vi "GetExcelWorkSheetIndexWithName.vi"(8 "error in":errorcluster, 11 "Path":path=path "O:/Monitor/m100schedule/history/1023MT人力配置AT機台排程.xls") -> (0 "error out":errorcluster, 2 "Sheets":string[](array[string]))   [LabVIEW 2012]
doc: "Before runnig this vi you need to select the sheet and the cell you want to retrieve in LabVIEW. When you start this vi, LabVIEW will ask you the name of the Excel file. This vi was written with Excel from MS Office 97. If you edit this VI and do not have this exact version of Excel registered correctly you will get a broken arrow due to the difference in ActiveX method among Excel version. Make sure you make a copy of this vi before editing it."
panel:
  out "index of element":i32
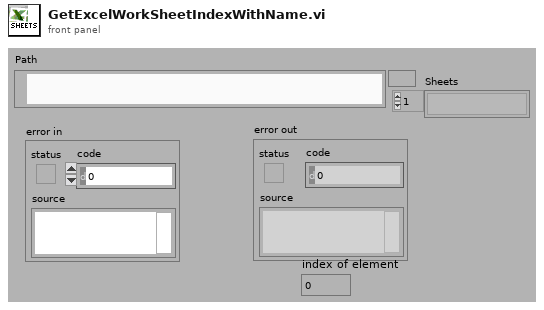
[diagram p1: front panel]
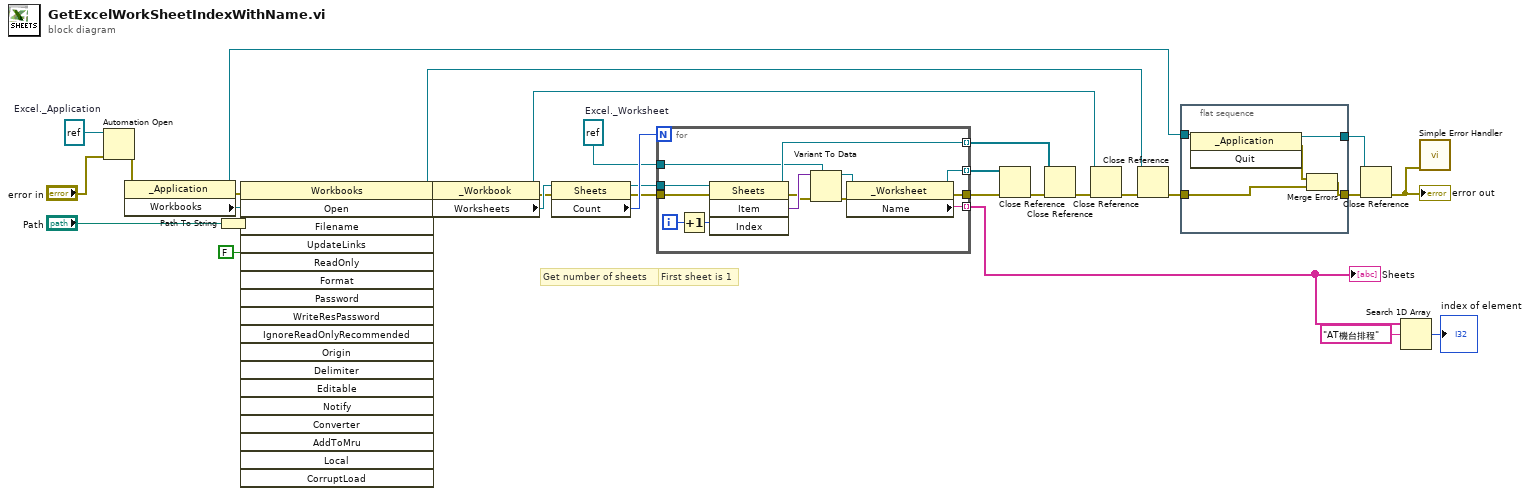
[diagram p0: block diagram]
diagram:
  w6 = refnum<k7> refnum  # Excel._Worksheet
  w20 = refnum<k7> refnum  # Excel._Application
  # "First sheet is 1"
  # "Get number of sheets"
  n1 = Automation Open(error in (no error)="error in", Automation Refnum=w20) -> (Automation Refnum=w29:refnum<k7>, error out=w33:errorcluster)  [unwired: 2 in]
  n2 = property class="_Application"(reference=w29, error in=w33) -> (reference out=w24:refnum<k7>, error out=w32:errorcluster, "Workbooks"=w18:refnum<k7>)
  n3 = Path To String(path="Path") -> (string=w31:string)
  n4 = invoke class="Workbooks" method="Open"(reference=w18, error in=w32, "Filename"=w31, "ReadOnly"=FALSE) -> (reference out=w19:refnum<k7>, error out=w14:errorcluster, "Open"=w17:refnum<k7>)  [unwired: 14 in, 15 out]
  n5 = property class="_Workbook"(reference=w17, error in=w14) -> (reference out=w5:refnum<k7>, error out=w13:errorcluster, "Worksheets"=w16:refnum<k7>)
  n6 = property class="Sheets"(reference=w16, error in=w13) -> (reference out=w12:refnum<k7>, error out=w11:errorcluster, "Count"=w15:i32)
  n7 = for {
    N: w15 -> [_]
    tunnel: [w41] -> w3 mode=indexing
    tunnel: [w42] -> w8
    tunnel: w12 -> [w39]
    tunnel: w11 -> [w38]
    tunnel: [w37] -> w10 mode=indexing
    tunnel: [w36] -> w9 mode=indexing
    tunnel: w6 -> [w34]
    i -> [w43]
    n8 = Increment(x=w43) -> (x+1=w40:i32)
    n9 = invoke class="Sheets" method="Item"(reference=w39, error in=w38, "Index"=w40) -> (reference out=w37:refnum<k7>, error out=w45:errorcluster, "Item"=w46:variant)  [unwired: 1 in, 1 out]
    n10 = Variant To Data(error in=w45, type=w34, Variant=w46) -> (data=w35:refnum<k7>, error out=w44:errorcluster)
    n11 = property class="_Worksheet"(reference=w35, error in=w44) -> (reference out=w36:refnum<k7>, error out=w42:errorcluster, "Name"=w41:string)
  }
  "Sheets" <- w3
  n12 = Close Reference(reference=w9, error in (no error)=w8) -> (error out=w28:errorcluster)
  n13 = Close Reference(reference=w10, error in (no error)=w28) -> (error out=w4:errorcluster)
  n14 = Close Reference(reference=w5, error in (no error)=w4) -> (error out=w27:errorcluster)
  n15 = Close Reference(reference=w19, error in (no error)=w27) -> (error out=w26:errorcluster)
  n16 = flat-sequence {
    tunnel: w26 -> [w47]
    tunnel: [w48] -> w25
    tunnel: w24 -> [w51]
    tunnel: [w50] -> w23
    frame #0 {
      n17 = invoke class="_Application" method="Quit"(reference=w51) -> (reference out=w50:refnum<k7>, error out=w49:errorcluster)  [unwired: 2 in, 1 out]
      n18 = Merge Errors(w49, w47) -> (w48:errorcluster)
    }
  }
  n19 = Close Reference(reference=w23, error in (no error)=w25) -> (error out=w22:errorcluster)
  "error out" <- w22
  n20 = Search 1D Array(1D array=w3, element="AT機台排程") -> (index of element=→"index of element":i32)  [unwired: 1 in]
  n21 = call <vilib>:"Simple Error Handler.vi"("error in (no error)"=w22) -> ()  [unwired: 4 in, 5 out]
